vi "Accumulated Angle.vi"() -> ()   [LabVIEW 2015]
panel:
  out "Calculated Angle":dbl
  in  "Gauge":dbl(knob) scale=0.0..360.0
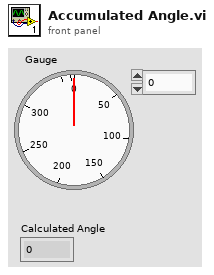
[diagram p1: front panel]
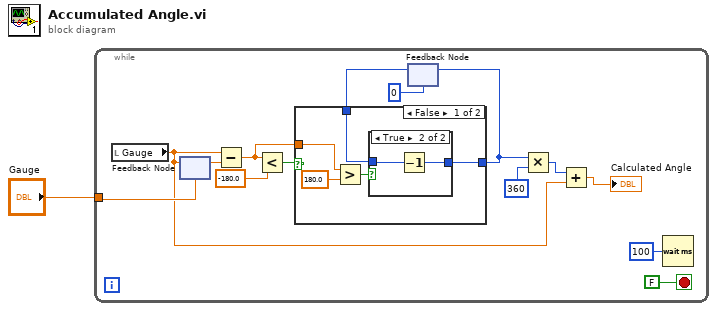
[diagram p0: block diagram]
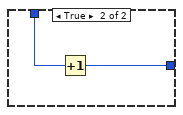
[diagram p3: hidden frame]
diagram:
  n1 = while {
    tunnel: "Gauge" -> [w4]
    stop <- FALSE stop-if-true
    n2 = local read "Gauge"() -> (w2:dbl)
    n3 = feedback-in #1(w2) -> ()
    n4 = feedback #1(w4) -> (w14:dbl)
    n5 = Subtract(x=w2, y=w14) -> (x-y=w8:dbl)
    n6 = Less?(x=w8, y=-180.0) -> (x < y?=w12:bool)
    n7 = feedback #2(0) -> (w9:i32)
    n8 = case shown="False" w12 {
      tunnel: [w16 w25] -> w7
      tunnel: w9 -> [w17 w24]
      tunnel: w8 -> [w20 _]
      frame False {
        n9 = Greater?(x=w20, y=180.0) -> (0:w18:bool)
        n10 = case shown="True" w18 {
          tunnel: w17 -> [w21 w23]
          tunnel: [w21 w22] -> w16
          frame False {
          }
          frame True {
            n11 = Decrement(x=w23) -> (x-1=w22:i32)
          }
        }
      }
      frame True {
        n12 = Increment(x=w24) -> (x+1=w25:i32)
      }
    }
    n13 = feedback-in #2(w7) -> ()
    n14 = Multiply(x=w7, y=360) -> (x*y=w5:i32)
    n15 = Add(x=w5, y=w2) -> (x+y=→"Calculated Angle":dbl)
    n16 = Wait (ms)(milliseconds to wait=u32 100) -> ()  [unwired: 1 out]
  }
